vi "SerializeToFile.vi"(8 "error in (no error)":errorcluster, 11 "FileConverterBase in":refnum<class "FileConverterBase.lvclass">) -> (0 "error out":errorcluster, 3 "FileConverterBase out":refnum<class "FileConverterBase.lvclass">)   [LabVIEW 2017, in "FileConverterBase.lvclass"]
uses:
  FileConverterBase.lvclass
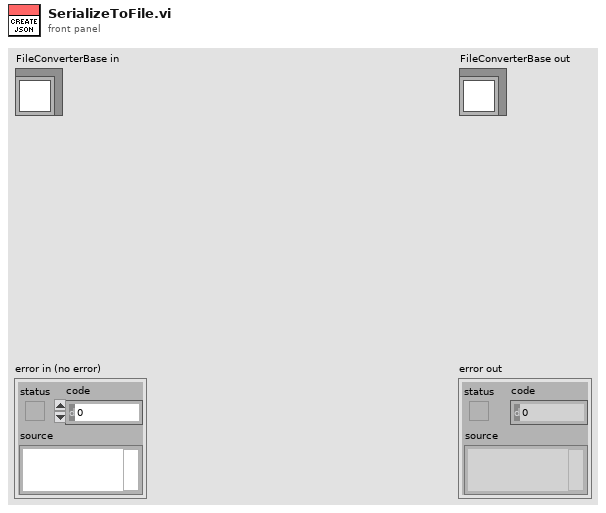
[diagram p1: front panel]
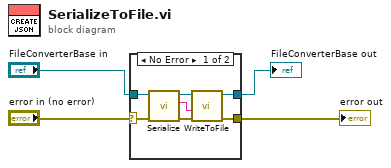
[diagram p0: block diagram]
diagram:
  n1 = case shown="No Error" "error in (no error)" {
    selector: "error in (no error)" -> [w6 w13]
    tunnel: [w5 w13] -> w3
    tunnel: [w9 w12] -> w1
    tunnel: "FileConverterBase in" -> [w11 w12]
    frame No Error {
      n2 = call-dynamic "Serialize.vi"("error in (no error)"=w6, "ConverterBase in"=w11) -> ("error out"=w7:errorcluster, "JSON"=w8:string, "ConverterBase out"=w10:refnum<class "FileConverterBase.lvclass">)  [unwired: 7 in]
      n3 = call-dynamic "WriteToFile.vi"("error in (no error)"=w7, "Serialized JSON"=w8, "ConverterBase in"=w10) -> ("error out"=w5:errorcluster, "ConverterBase out"=w9:refnum<class "FileConverterBase.lvclass">)  [unwired: 7 in]
    }
    frame Error {
    }
  }
  "error out" <- w3
  "FileConverterBase out" <- w1
